vi "Load IBW File.vi"(2 "Page":i32, 3 "file path (dialog if empty)":path=path "C:/Work/IBW - LVArray/BTOCu1005.ibw") -> (0 "Image":T1(plugin-control), 1 "Wave Note":string)   [LabVIEW 2011]
uses:
  <vilib>/vision/NI_Vision_Development_Module.lvlib
panel:
  out "error out":errorcluster
  in  "Type of Symmetry":u32(ring) items=["Horizontal", "Vertical", "Central", "1st Diagonal", "2nd Diagonal"]
  out "Wave Name":string
  in  "Array":i8[](array[numeric])
  out "Wave Created":timestamp format="%<%.3X\n%Y/%m/%d>T"
  in  "dates and points":T2
  in  "Array 2":i8[](array[numeric])
  out "Output Array":dbl[][][](array[numeric])
  out "Intensity Graph":sgl[][](graph)
  in  "Cluster":T3
  out "dim size":i32[](array[numeric])
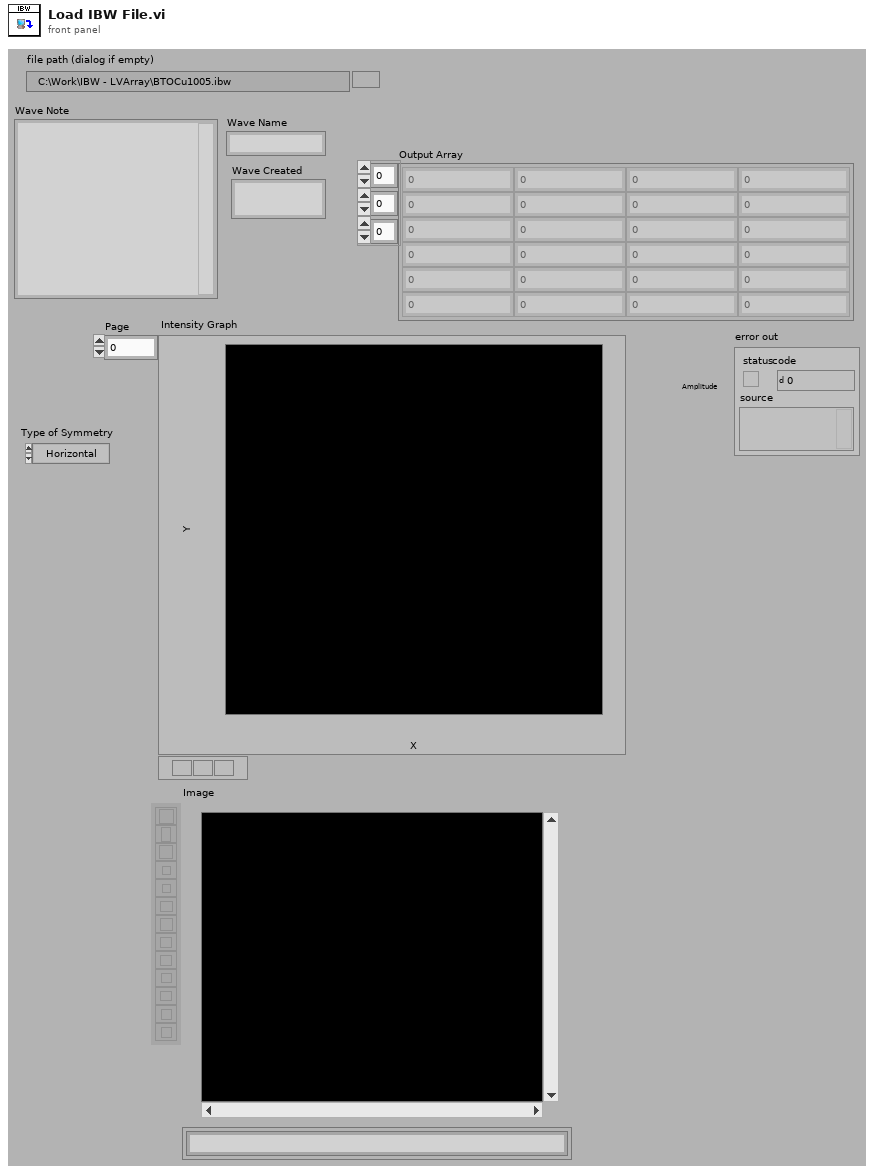
[diagram p1: front panel]
types:
  T1 = typedef "IMAQ Image.ctl" = refnum<image>
  T2 = cluster{"creation date":u32, "mod date":u32, "nmpnts":i32, "type":i16}
  T3 = cluster{"version":i16, "checksum":i16, "wfmSize":i32, "formulaSize":i32, "noteSize":i32}
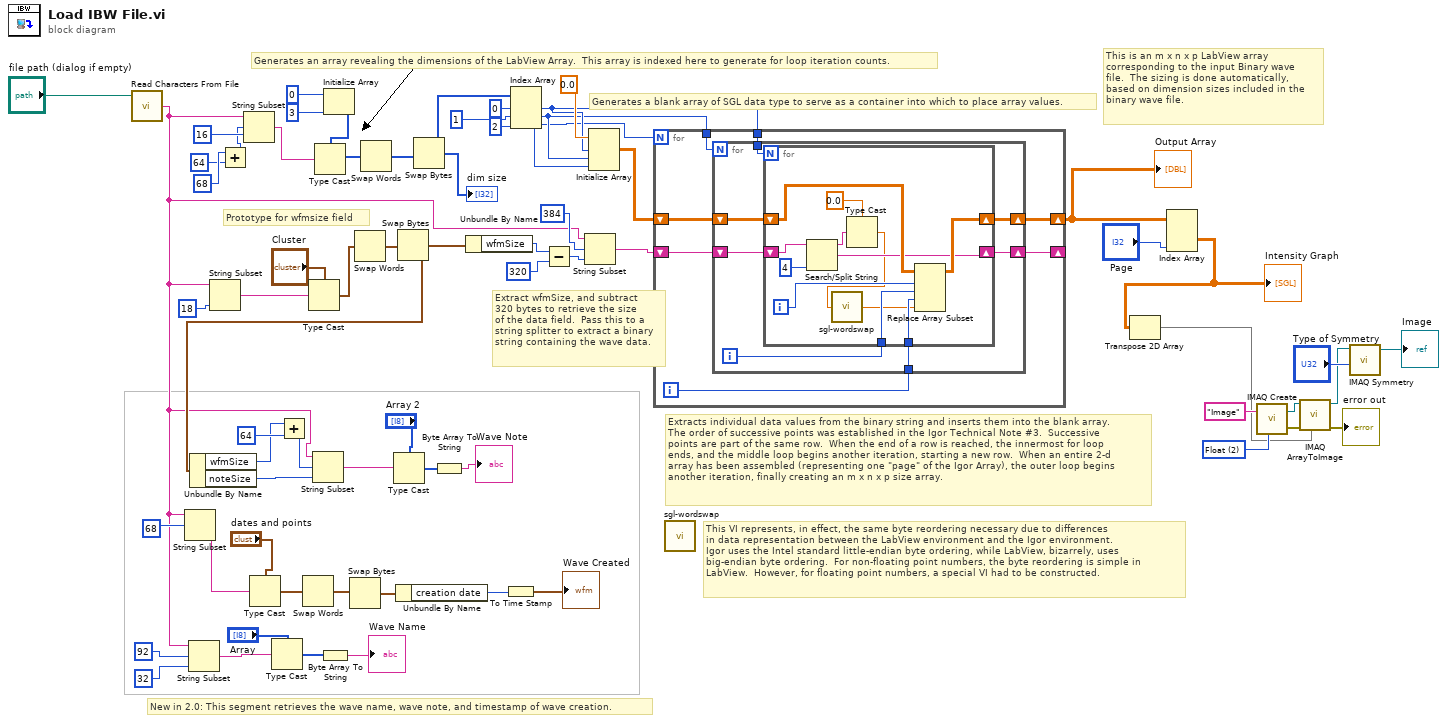
[diagram p0: block diagram]
diagram:
  w6 = u32 2 items=["8 bits", "16 bits", "Float", "Complex", "RGB", "HSL"] ("Image Type")
  # "New in 2.0: This segment retrieves the wave name, wave note, and timestamp of wave creation."
  # "This VI represents, in effect, the same byte reordering necessary due to differences\nin data representation between the LabView environment and the Igor environment.\nIgor uses the Intel standard little-endian byte ordering, while LabView, bizarrely, uses\nbig-endian byte ordering.  For non-floating point numbers, the byte reordering is simple in\nLabView.  However, for floating point numbers, a special VI had to be constructed."
  # "This is an m x n x p LabView array\ncorresponding to the input Binary wave\nfile.  The sizing is done automatically,\nbased on dimension sizes included in the\nbinary wave file."
  # "Generates a blank array of SGL data type to serve as a container into which to place array values."
  # "Extracts individual data values from the binary string and inserts them into the blank array.\nThe order of successive points was established in the Igor Technical Note #3.  Successive\npoints are part of the same row.  When the end of a row is reached, the innermost for loop\nends, and the middle loop begins another iteration, starting a new row.  When an entire 2-d\narray has been assembled (representing one \"page\" of the Igor Array), the outer loop begins\nanother iteration, finally creating an m x n x p size array."
  # "Extract wfmSize, and subtract\n320 bytes to retrieve the size\nof the data field.  Pass this to a\nstring splitter to extract a binary\nstring containing the wave data."
  # "Prototype for wfmsize field"
  # "Generates an array revealing the dimensions of the LabView Array.  This array is indexed here to generate for loop iteration counts."
  n1 = call <vilib>:"Read Characters From File.vi"("file path (dialog if empty)"="file path (dialog if empty)") -> ("character string"=w11:string)  [unwired: 1 in, 7 out]
  n2 = String Subset(string=w11, offset (0)=68 ("nmpnts offset")) -> (substring=w24:string)  [unwired: 1 out]
  n3 = String Subset(string=w11, offset (0)=92 ("wave name offset"), length (rest)=32 ("length (rest)")) -> (substring=w15:string)
  n4 = String Subset(string=w11, length (rest)=18 ("length (rest)")) -> (substring=w58:string)  [unwired: 1 out]
  n5 = Add(x=68 ("dims offset"), y=64) -> (x+y=w44:i32)
  n6 = String Subset(string=w11, offset (0)=w44, length (rest)=16 ("length (rest)")) -> (substring=w63:string)
  n7 = Type Cast(type="dates and points", x=w24) -> (*(type *) &x=w19:T2)
  n8 = Type Cast(type="Array", x=w15) -> (*(type *) &x=w13:i8[])
  n9 = Swap Words(1:w19) -> (0:w18:T2)
  n10 = Type Cast(type="Cluster", x=w58) -> (*(type *) &x=w30:T3)
  n11 = Byte Array To String(unsigned byte array=w13) -> (string=→"Wave Name":string)
  n12 = Initialize Array(0 ("element"), 3 ("dimension size")) -> (w64:i32[])
  n13 = Type Cast(type=w64, x=w63) -> (*(type *) &x=w65:i32[])
  n14 = Swap Bytes(anything=w18) -> (byte swapped=w22:T2)
  n15 = Swap Words(1:w30) -> (0:w60:T3)
  n16 = Swap Words(1:w65) -> (0:w66:i32[])
  n17 = Unbundle By Name(w22) -> ("creation date"=w20:u32)
  n18 = Swap Bytes(anything=w60) -> (byte swapped=w28:T3)
  n19 = Unbundle By Name(w28) -> ("wfmSize"=w27:i32, "noteSize"=w26:i32)
  n20 = Add(x=w27, y=64) -> (x+y=w34:i32)
  n21 = String Subset(string=w11, offset (0)=w34, length (rest)=w26) -> (substring=w33:string)
  n22 = Type Cast(type="Array 2", x=w33) -> (*(type *) &x=w31:i8[])
  n23 = Swap Bytes(anything=w66) -> (byte swapped=w52:i32[])
  "dim size" <- w52
  n24 = Byte Array To String(unsigned byte array=w31) -> (string=→"Wave Note":string)
  n25 = Unbundle By Name(w28) -> ("wfmSize"=w56:i32)
  n26 = To Time Stamp(1:w20) -> (0:→"Wave Created":timestamp)
  n27 = Index Array(array=w52, index #1=0 ("index"), index #2=1 ("index"), index #3=2 ("index")) -> (element #1=w39:i32, element #2=w38:i32, element #3=w37:i32)
  n28 = Subtract(x=w56, y=320) -> (x-y=w54:i32)
  n29 = String Subset(string=w11, offset (0)=384, length (rest)=w54) -> (substring=w41:string)
  n30 = Initialize Array(sgl 0.0 ("element"), w39, w38, w37) -> (w48:sgl[][][])
  n31 = for {
    N: w37 -> [_]
    shift-right: [w69] -> w47
    shift-left: w48 -> [w73]
    shift-right: [w68] -> _
    shift-left: w41 -> [w72]
    tunnel: w39 -> [w71]
    tunnel: w38 -> [w67]
    i -> [w70]
    n32 = for {
      N: w67 -> [_]
      shift-right: [w75] -> w69
      shift-left: w73 -> [w80]
      shift-right: [w74] -> w68
      shift-left: w72 -> [w79]
      tunnel: w71 -> [w78]
      tunnel: w70 -> [w76]
      i -> [w77]
      n33 = for {
        N: w78 -> [_]
        shift-right: [w86] -> w75
        shift-left: w80 -> [w90]
        shift-right: [w85] -> w74
        shift-left: w79 -> [w91]
        tunnel: w77 -> [w88]
        tunnel: w76 -> [w87]
        i -> [w89]
        n34 = Search/Split String(string=w91, offset (0)=4 ("length (rest)")) -> (substring before match=w84:string, match + rest of string=w85:string)  [unwired: 2 out]
        n35 = Type Cast(type=sgl 0.0, x=w84) -> (*(type *) &x=w82:sgl)
        n36 = call <userlib>:"sgl-wordswap.vi"("x"=w82) -> ("*(type *) &x"=w81:sgl)
        n37 = Replace Array Subset(array=w90, new element=w81, index (dim 0)=w89, index (dim 1)=w88, index (dim 2)=w87) -> (w86:sgl[][][])
      }
    }
  }
  "Output Array" <- w47
  n38 = call <userlib>:"sgl-wordswap.vi"() -> ()  [unwired: 1 in, 1 out]
  n39 = Index Array(array=w47, index (dim 2)="Page") -> (element=w10:sgl[][])  [unwired: 2 in]
  "Intensity Graph" <- w10
  n40 = Transpose 2D Array(2D array=w10) -> (transposed array=w1:sgl[][])
  n41 = call "IMAQ Create"("Image Name"="Image", "Image Type"=w6) -> ("New Image"=w7:T1, "error out"=w5:errorcluster)  [unwired: 2 in, 1 out]
  n42 = call "IMAQ ArrayToImage"("Image Pixels (Float)"=w1, "error in (no error)"=w5, "Image"=w7) -> ("error out"=→"error out":errorcluster, "Image Out"=w3:T1)  [unwired: 3 in, 4 out]
  n43 = call "IMAQ Symmetry"("Type of Symmetry"="Type of Symmetry", "Image Src"=w3) -> ("Image Dst Out"=→"Image":T1)  [unwired: 2 in, 2 out]
